vi "Baseline Value at X.vi"(4 "min points to fit (100)":i32=100, 6 "num segments before":i32, 7 "X":dbl format="%.2f", 8 "baseline Y[]":dbl[](array[numeric]) format="%.2f", 9 "baseline X[]":dbl[](array[numeric]) format="%.2f") -> (0 "num segments after":i32, 1 "Y":dbl format="%.2f", 2 "baseline Y[]":dbl[](array[numeric]) format="%.2f", 3 "baseline X[]":dbl[](array[numeric]) format="%.2f")   [LabVIEW 2012]
doc: "Calculates the Y value of the baseline at the given X (time) from the last non-empty segment of the baseline X and Y arrays. The baseline is composed of 'num segments' linear segments, defined by two XY points each, and zero or more points following those that define the current segment. If the current segment has at least 'min points to fit' points, then they are replaced in the output baseline arrays with two points found by a linear fit.\n\nUse the help window to read the descriptions of the individual controls for more information about this VI's inputs and outputs."
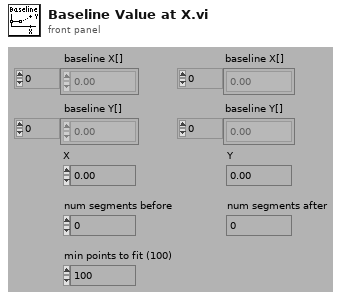
[diagram p1: front panel]
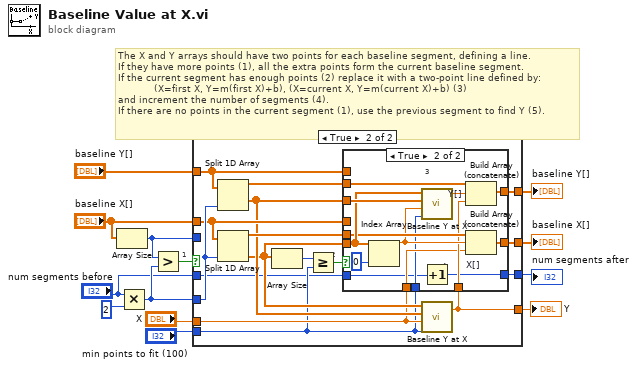
[diagram p0: block diagram]
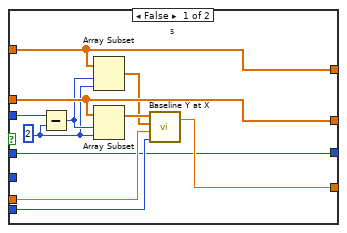
[diagram p2: hidden frame]
diagram:
  # "1"
  # "The X and Y arrays should have two points for each baseline segment, defining a line.\nIf they have more points (1), all the extra points form the current baseline segment.\nIf the current segment has enough points (2) replace it with a two-point line defined by:\n            (X=first X, Y=m(first X)+b), (X=current X, Y=m(current X)+b) (3)\nand increment the number of segments (4).\nIf there are no points in the current segment (1), use the previous segment to find Y (5)."
  n1 = Array Size(array="baseline X[]") -> (size(s)=w5:i32)
  n2 = Multiply(x="num segments before", y=2) -> (x*y=w11:i32)
  n3 = Greater?(x=w5, y=w11) -> (0:w9:bool)
  n4 = case shown="True" w9 {
    tunnel: "baseline X[]" -> [w23 w34]
    tunnel: w11 -> [_ w40]
    tunnel: "baseline Y[]" -> [w22 w35]
    tunnel: "X" -> [w17 w29]
    tunnel: [w22 w37] -> w7
    tunnel: [w23 w36] -> w6
    tunnel: w5 -> [w24 _]
    tunnel: "min points to fit (100)" -> [w16 w27]
    tunnel: [w15 w30] -> w3
    tunnel: "num segments before" -> [w14 w26]
    tunnel: [w14 w25] -> w1
    frame False {
      w20 = 2
      # "5"
      n5 = Subtract(x=w24, y=w20) -> (x-y=w21:i32)
      n6 = Array Subset(array=w22, index=w21, length=w20) -> (w18:dbl[])
      n7 = Array Subset(array=w23, index=w21, length=w20) -> (w19:dbl[])
      n8 = call "Baseline Y at X.vi"("min points to fit (100)"=w16, "X"=w17, "baseline Y[]"=w18, "baseline X[]"=w19) -> ("Y"=w15:dbl)  [unwired: 1 in]
    }
    frame True {
      # "2"
      n9 = Split 1D Array(array=w35, index=w40) -> (first subarray=w39:dbl[], second subarray=w32:dbl[])
      n10 = Split 1D Array(array=w34, index=w40) -> (first subarray=w38:dbl[], second subarray=w31:dbl[])
      n11 = Array Size(array=w31) -> (size(s)=w33:i32)
      n12 = Greater Or Equal?(x=w33, y=w27) -> (x >= y?=w28:bool)
      n13 = call "Baseline Y at X.vi"("min points to fit (100)"=w27, "X"=w29, "baseline Y[]"=w32, "baseline X[]"=w31) -> ("Y"=w30:dbl)  [unwired: 1 in]
      n14 = case shown="True" w28 {
        tunnel: w39 -> [_ w55]
        tunnel: w38 -> [_ w51]
        tunnel: w31 -> [_ w53]
        tunnel: [w42 w56] -> w37
        tunnel: [w43 w47] -> w36
        tunnel: w35 -> [w42 _]
        tunnel: w34 -> [w43 _]
        tunnel: w32 -> [_ w54]
        tunnel: w30 -> [_ w49]
        tunnel: w29 -> [_ w48]
        tunnel: w27 -> [_ w46]
        tunnel: w26 -> [w41 w45]
        tunnel: [w41 w44] -> w25
        frame False {
        }
        frame True {
          # "4"
          # "3"
          n15 = Index Array(array=w53, index=0) -> (element=w50:dbl)
          n16 = call "Baseline Y at X.vi"("min points to fit (100)"=w46, "X"=w50, "baseline Y[]"=w54, "baseline X[]"=w53) -> ("Y"=w52:dbl)  [unwired: 1 in]
          n17 = Increment(x=w45) -> (x+1=w44:i32)
          n18 = Build Array (concatenate) "Y[]"(w55, w52, w49) -> (w56:dbl[])
          n19 = Build Array (concatenate) "X[]"(w51, w50, w48) -> (w47:dbl[])
        }
      }
    }
  }
  "baseline X[]" <- w6
  "baseline Y[]" <- w7
  "Y" <- w3
  "num segments after" <- w1
